vi "TurretSetpointSelect.vi"(4 "TurretManualControlActive":bool, 5 "ManualSetpointEnable":bool, 6 "CurrentTurretPosition(deg)":dbl, 7 "ManualSetpointActivate":bool, 8 "VisionTarget":T1, 9 "limelight_set_point":dbl, 10 "AutoTargetActivate":bool, 11 "ManualSetpoint(deg)":dbl) -> (1 "Setpoint(deg)":dbl, 2 "ActivateAutoControl":bool)   [LabVIEW 2019]
uses:
  Vision/TypeDefs/VisionTarget.ctl
  ArgosLib/Signal Processing/TypeDefs/EdgeDetector_Type.ctl
  ArgosLib/ArgosLib.lvlib
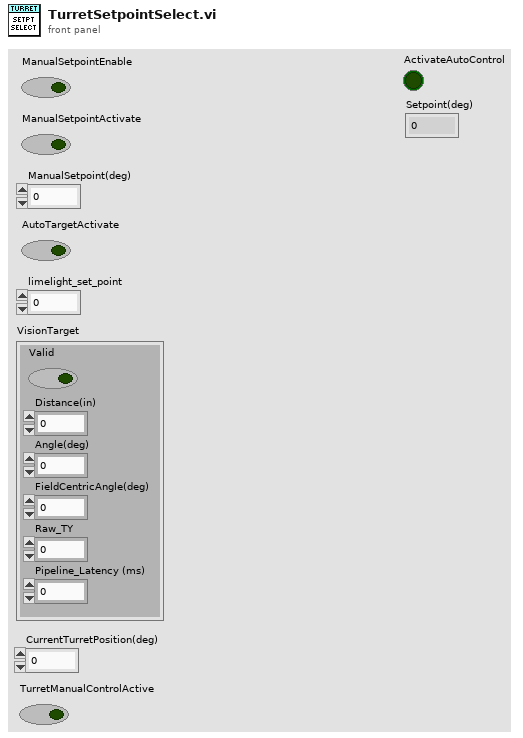
[diagram p1: front panel]
types:
  T1 = typedef "VisionTarget.ctl" = cluster{"Valid":bool, "Distance(in)":dbl, "Angle(deg)":dbl, "FieldCentricAngle(deg)":dbl, "Raw_TY":dbl, "Pipeline_Latency (ms)":dbl}
  T2 = typedef "ArgosLib.lvlib/EdgeDetector_Type.ctl" = enum16{"RisingEdge", "FallingEdge", "Both"}
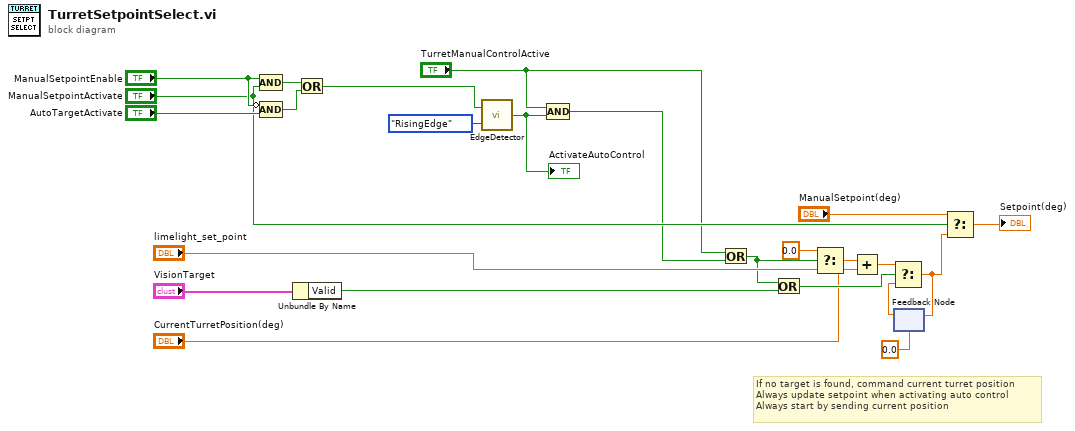
[diagram p0: block diagram]
diagram:
  # "If no target is found, command current turret position\nAlways update setpoint when activating auto control\nAlways start by sending current position"
  n1 = Compound Arithmetic op=AND("ManualSetpointEnable", "ManualSetpointActivate") -> (w23:bool)
  n2 = Compound Arithmetic op=AND(invert "ManualSetpointEnable", "AutoTargetActivate") -> (w22:bool)
  n3 = Unbundle By Name("VisionTarget") -> ("Valid"=w10:bool)
  n4 = Or(x=w23, y=w22) -> (x .or. y?=w21:bool)
  n5 = call "EdgeDetector.vi"("DetectorType"=EdgeDetector_Type."RisingEdge", "Input"=w21) -> ("Edge"=w5:bool)
  "ActivateAutoControl" <- w5
  n6 = Compound Arithmetic op=AND("TurretManualControlActive", w5) -> (w2:bool)
  n7 = Or(x="TurretManualControlActive", y=w2) -> (x .or. y?=w1:bool)
  n8 = Or(x=w1, y=w10) -> (x .or. y?=w11:bool)
  n9 = Select(t=0.0, s=w1, f="limelight_set_point") -> (s? t:f=w13:dbl)
  n10 = Add(x=w13, y="CurrentTurretPosition(deg)") -> (x+y=w15:dbl)
  n11 = feedback #1(0.0) -> (w16:dbl)
  n12 = Select(t=w15, s=w11, f=w16) -> (s? t:f=w14:dbl)
  n13 = feedback-in #1(w14) -> ()
  n14 = Select(t="ManualSetpoint(deg)", s="ManualSetpointActivate", f=w14) -> (s? t:f=→"Setpoint(deg)":dbl)
